vi "ShutDownServer.vi"() -> ()   [LabVIEW 2011]
panel:
  out "ShutDownServer":bool
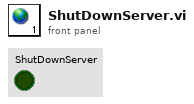
[diagram p1: front panel]
diagram:
